vi "AddorEdit Devicetype Variable.vi"(0 "Device Name":string, 5 "<Settings Selected elements SET=NO>":string[](array[string]), 7 "Settings variant":variant, 9 "Subscriber Variant":variant, 11 "error in":errorcluster, 12 "Devicetype \nvariable Units":string[][](array[string])) -> (4 "Devicetype variable list":string[][](array[string]), 15 "error out":errorcluster)   [LabVIEW 2020]
panel:
  out "Array":string[][](array[string])
  out "Devicetype Variable \nData":string[][](array[string])
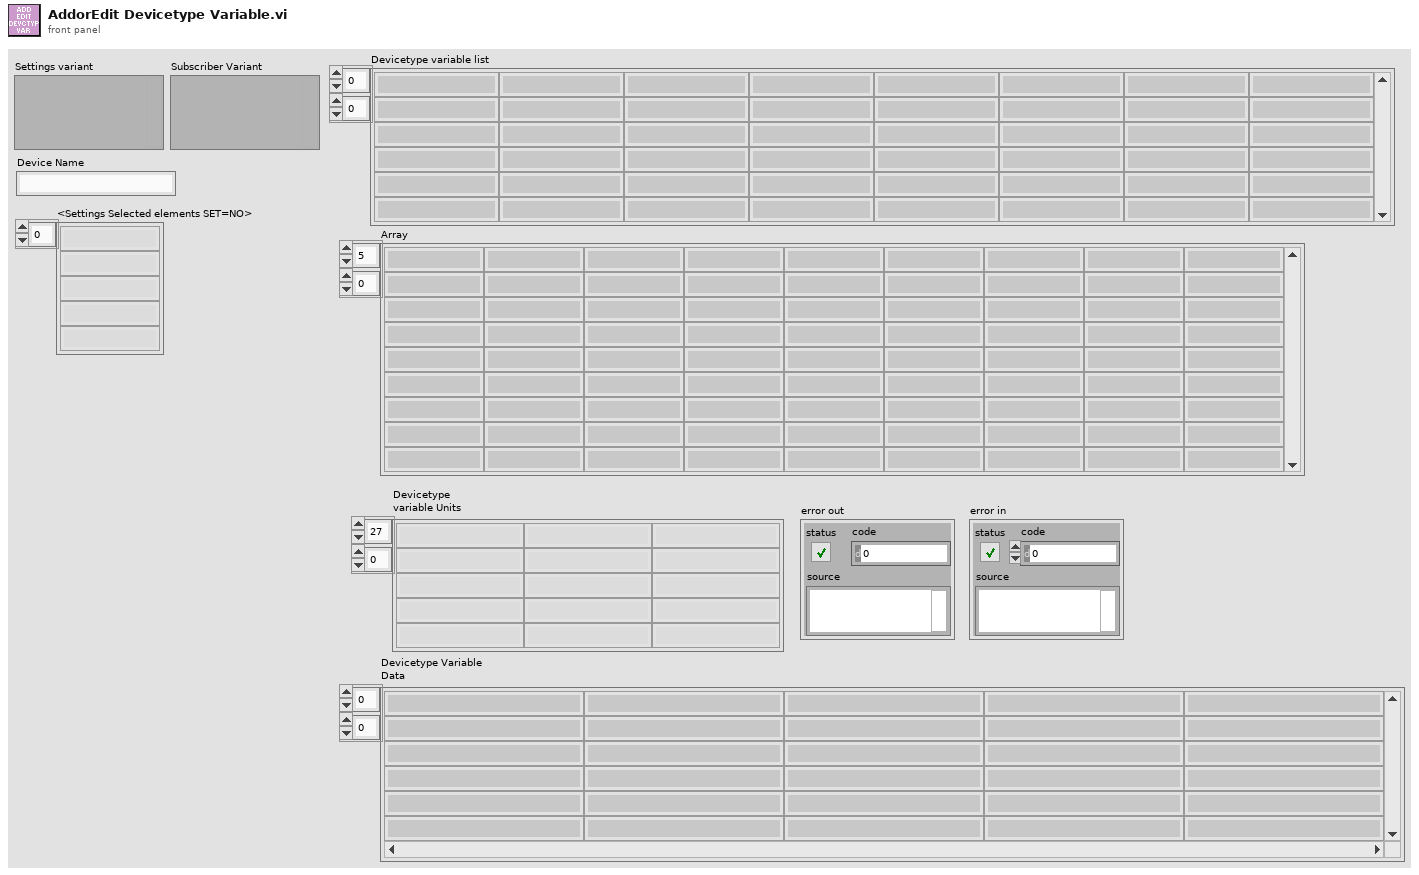
[diagram p1: front panel]
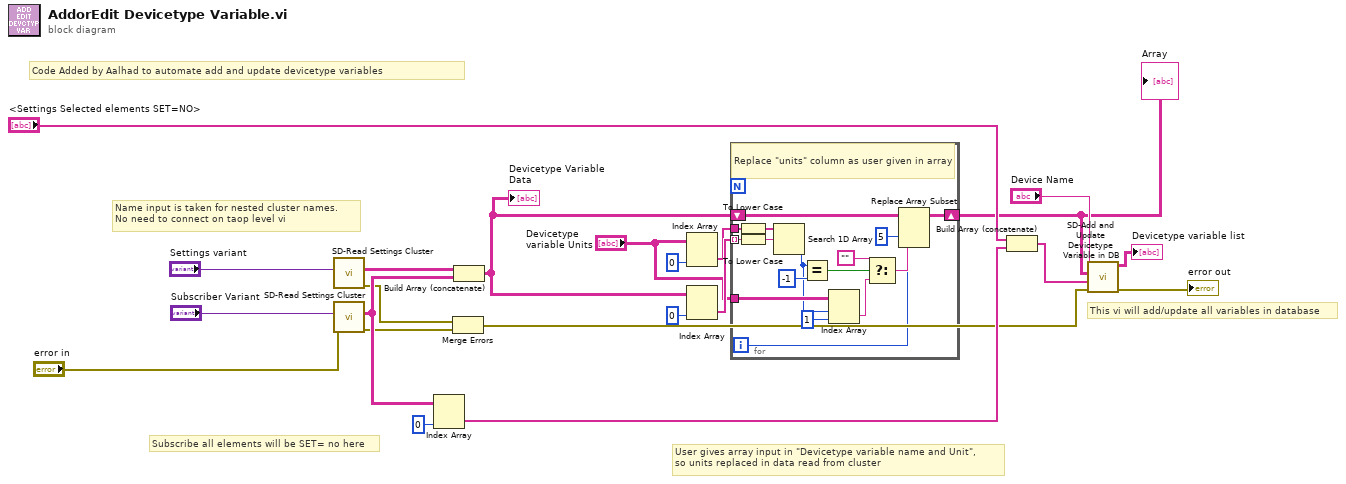
[diagram p0: block diagram]
diagram:
  # "User gives array input in \"Devicetype variable name and Unit\", \nso units replaced in data read from cluster"
  # "Name input is taken for nested cluster names. \nNo need to connect on taop level vi"
  # "This vi will add/update all variables in database"
  # "Subscribe all elements will be SET= no here"
  # "Code Added by Aalhad to automate add and update devicetype variables"
  n1 = call "SD-Read Settings Cluster.vi"("variant"="Settings variant") -> ("error out"=w14:errorcluster, "Devicetype Variable \nData"=w13:string[][])  [unwired: 9 in]
  n2 = call "SD-Read Settings Cluster.vi"("error in"="error in", "variant"="Subscriber Variant") -> ("error out"=w15:errorcluster, "Devicetype Variable \nData"=w17:string[][])  [unwired: 8 in]
  n3 = Index Array(array=w17, index (col)=0 ("disabled index (col)")) -> (element=w20:string[])  [unwired: 1 in]
  n4 = Merge Errors(w14, w15) -> (w16:errorcluster)
  n5 = Build Array (concatenate)(w13, w17) -> (w1:string[][])
  "Devicetype Variable \nData" <- w1
  n6 = Index Array(array="Devicetype \nvariable Units", index (col)=0 ("disabled index (col)")) -> (element=w4:string[])  [unwired: 1 in]
  n7 = Index Array(array=w1, index (col)=0 ("index (row)")) -> (element=w7:string[])  [unwired: 1 in]
  n8 = for {
    tunnel: w7 -> [w38] mode=indexing
    tunnel: w4 -> [w37]
    tunnel: "Devicetype \nvariable Units" -> [w36]
    shift-right: [w33] -> w2
    shift-left: w1 -> [w34]
    i -> [w25]
    # "Replace \"units\" column as user given in array"
    n9 = To Lower Case(string=w37) -> (all lower case string=w24:string[])
    n10 = To Lower Case(string=w38) -> (all lower case string=w23:string)
    n11 = Search 1D Array(1D array=w24, element=w23) -> (index of element=w31:i32)  [unwired: 1 in]
    n12 = Equal?(x=w31, y=-1 ("disabled index (col)")) -> (x = y?=w29:bool)
    n13 = Index Array(array=w36, index (row)=w31, index (col)=1 ("disabled index (col)")) -> (element=w28:string)
    n14 = Select(t="", s=w29, f=w28) -> (s? t:f=w26:string)
    n15 = Replace Array Subset(array=w34, new element=w26, index (row)=w25, index (col)=5 ("disabled index (col)")) -> (w33:string[][])
  }
  "Array" <- w2
  n16 = Build Array (concatenate)("<Settings Selected elements SET=NO>", w20) -> (w22:string[])
  n17 = call "SD-Add and Update Devicetype Variable in DB.vi"("error in"=w16, "Dont Set variables list"=w22, "Devicetype variable\nCluster Data"=w2, "Device Name"="Device Name") -> ("error out"=→"error out":errorcluster, "Devicetype \nvariable DB data"=→"Devicetype variable list":string[][])  [unwired: 6 in]
